vi "DT_Triangle Manager_Format Edge.vi"(9 "start triangle":i32, 10 "point 2":i32, 11 "point 1":i32) -> (2 "Second Triangle":i32[](array[numeric]), 3 "First Triangle":i32[](array[numeric]))   [LabVIEW 2020, in "NI_AAL_Geometry.lvlib"]
uses:
  <vilib>/Analysis/NI_AAL_Geometry.lvlib
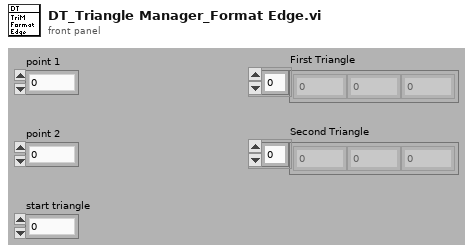
[diagram p1: front panel]
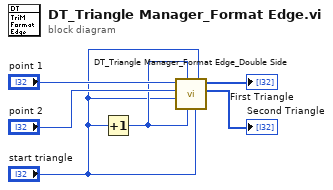
[diagram p0: block diagram]
diagram:
  n1 = Increment(x="start triangle") -> (x+1=w4:i32)
  n2 = call <vilib>:"DT_Triangle Manager_Format Edge_Double Side.vi"("right bottom tri"="start triangle", "left bottom tri"="start triangle", "right top tri"=w4, "left top tri"=w4, "start triangle"="start triangle", "right point"="point 2", "left point"="point 1") -> ("Second Triangle"=→"Second Triangle":i32[], "First Triangle"=→"First Triangle":i32[])  [unwired: 3 out]
